vi "__Init Cloud List Menu.vi"(8 "error in (no error)":errorcluster, 9 "MCListbox Refnum":refnum<vi>, 10 "Coords":T1, 11 "menu reference":refnum<k9>) -> (0 "error out":errorcluster, 3 "Discard?":bool)   [LabVIEW 2011]
doc: "Fills the right-click menu associated with the cloud list Multicolumn Listbox with the proper items, based on what kind of item the click happened on (file/folder/empty item)."
uses:
  <vilib>/Utility/miscctls.llb/LVPoint32TypeDef.ctl
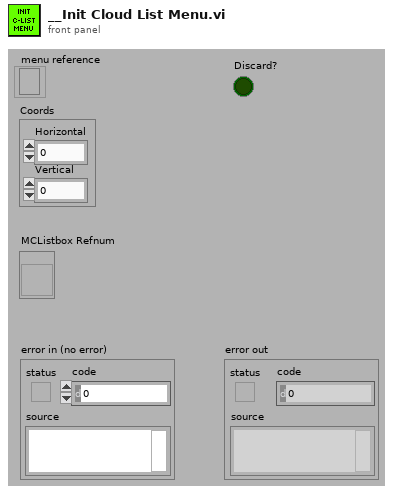
[diagram p1: front panel]
types:
  T1 = typedef "LVPoint32TypeDef.ctl" = cluster{"Horizontal":i32, "Vertical":i32}
  T2 = typedef "LVRowAndColumnTypeDef.ctl" = cluster{"Row":i32, "Column":i32}
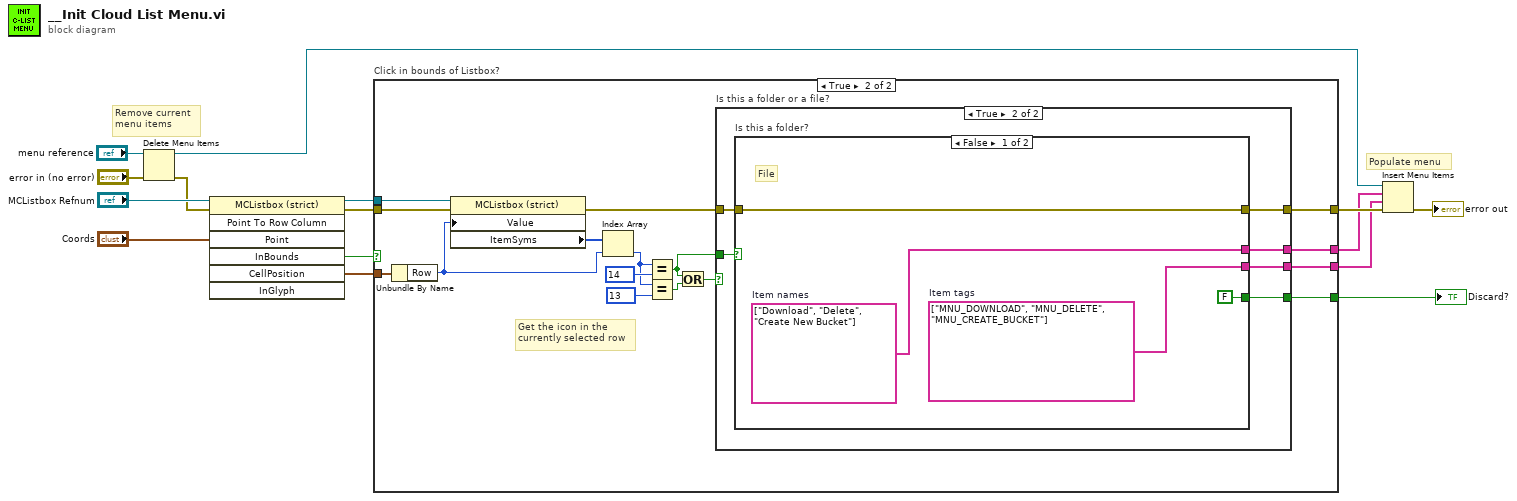
[diagram p0: block diagram]
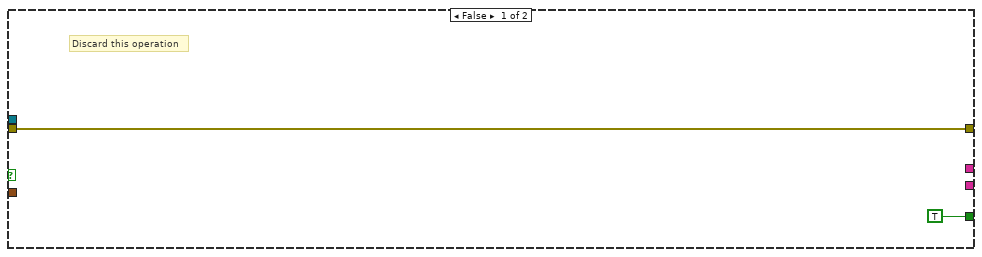
[diagram p2: hidden frame]
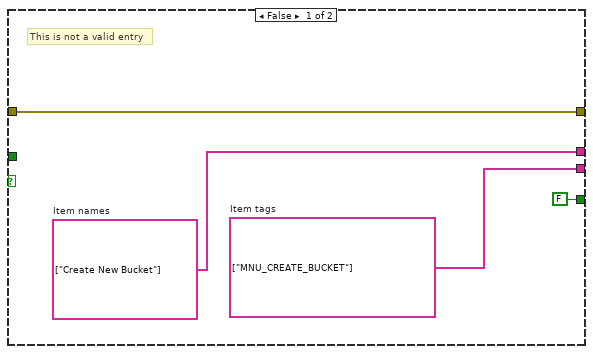
[diagram p3: hidden frame]
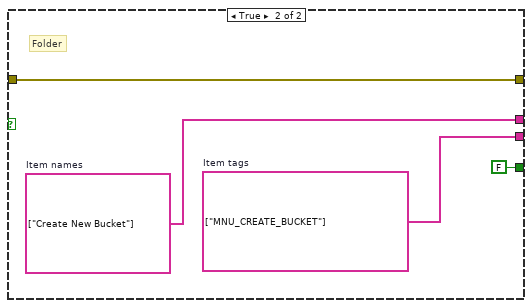
[diagram p4: hidden frame]
diagram:
  # "Populate menu"
  # "Remove current\nmenu items"
  n1 = Delete Menu Items(6:"error in (no error)", 9:"menu reference") -> (0:w11:errorcluster, 3:w3:refnum<k9>)  [unwired: 2 in]
  n2 = invoke class="MCListbox (strict)" method="Point To Row Column"(reference="MCListbox Refnum", error in=w11, "Point"="Coords") -> (reference out=w7:refnum<vi>, error out=w8:errorcluster, "InBounds"=w10:bool, "CellPosition"=w9:T2)  [unwired: 4 in, 3 out]
  n3 = case "Click in bounds of Listbox?" shown="True" w10 {
    tunnel: w9 -> [_ w33]
    tunnel: w8 -> [w17 w32]
    tunnel: w7 -> [_ w31]
    tunnel: [_ w22] -> w5
    tunnel: [_ w21] -> w4
    tunnel: [w17 w19] -> w6
    tunnel: [TRUE w18] -> w1
    frame False {
      # "Discard this operation"
    }
    frame True {
      # "Get the icon in the\ncurrently selected row"
      n4 = Unbundle By Name(w33) -> ("Row"=w29:i32)
      n5 = property class="MCListbox (strict)"(reference=w31, error in=w32, "Value"=w29) -> (error out=w20:errorcluster, "ItemSyms"=w30:i32[])  [unwired: 1 out]
      n6 = Index Array(array=w30, index=w29) -> (element=w26:i32)
      n7 = Equal?(x=w26, y=14) -> (x = y?=w23:bool)
      n8 = Equal?(x=w26, y=13) -> (x = y?=w25:bool)
      n9 = Or(x=w23, y=w25) -> (x .or. y?=w24:bool)
      n10 = case "Is this a folder or a file?" shown="True" w24 {
        tunnel: w23 -> [_ w43]
        tunnel: [w36 w42] -> w22
        tunnel: [w35 w41] -> w21
        tunnel: w20 -> [w37 w40]
        tunnel: [w37 w39] -> w19
        tunnel: [FALSE w38] -> w18
        frame False {
          w35 = string[] ["MNU_CREATE_BUCKET"]  # Item tags
          w36 = string[] ["Create New Bucket"]  # Item names
          # "This is not a valid entry"
        }
        frame True {
          n11 = case "Is this a folder?" shown="False" w43 {
            tunnel: [w47 w51] -> w42
            tunnel: [w46 w50] -> w41
            tunnel: w40 -> [w45 w49]
            tunnel: [w45 w49] -> w39
            tunnel: [FALSE FALSE] -> w38
            frame False {
              w46 = string[] ["MNU_DOWNLOAD", "MNU_DELETE", "MNU_CREATE_BUCKET"]  # Item tags
              w47 = string[] ["Download", "Delete", "Create New Bucket"]  # Item names
              # "File"
            }
            frame True {
              w50 = string[] ["MNU_CREATE_BUCKET"]  # Item tags
              w51 = string[] ["Create New Bucket"]  # Item names
              # "Folder"
            }
          }
        }
      }
    }
  }
  "Discard?" <- w1
  n12 = Insert Menu Items(6:w6, 7:w4, 8:w5, 9:w3) -> (0:→"error out":errorcluster)  [unwired: 2 in, 2 out]
